vi "Save Instance VI to Polymorphic (strange poly vim saving).vi"(8 "error in (no error)":errorcluster, 10 "Polymorphic Label":string, 11 "SubVI Ref In":refnum<vi>) -> (0 "error out":errorcluster, 3 "Polymorphic VI":path)   [LabVIEW 2020]
uses:
  <vilib>/LabVIEW Icon API/LabVIEW Icon API.lvlib
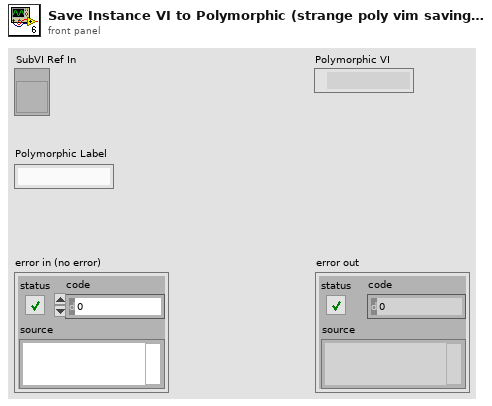
[diagram p1: front panel]
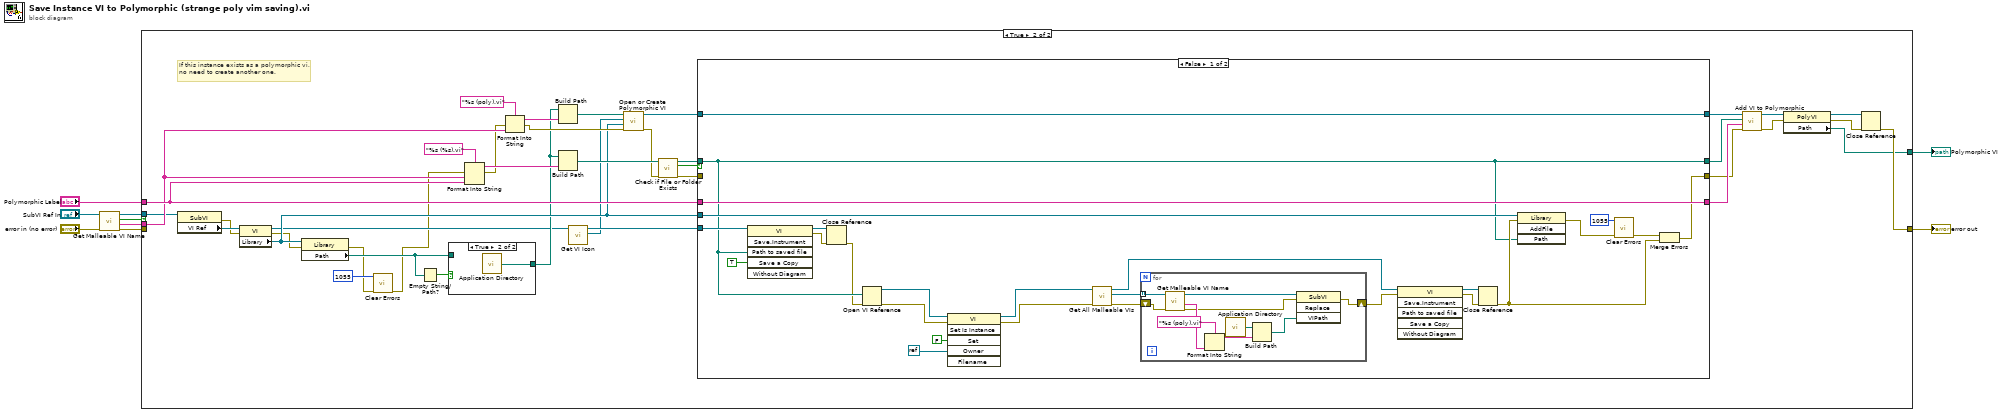
[diagram p0: block diagram]
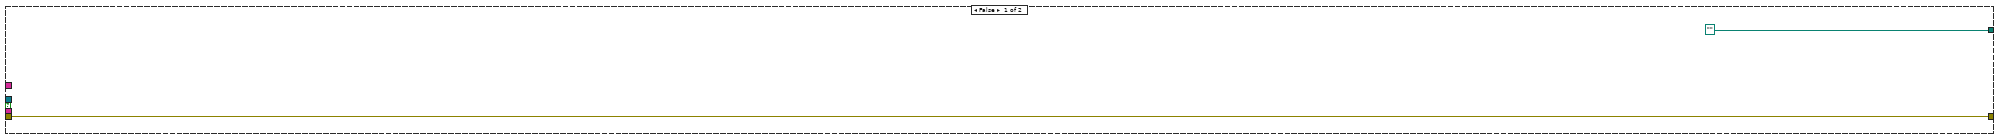
[diagram p2: hidden frame]
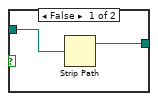
[diagram p3: hidden frame]
diagram:
  n1 = call "Get Malleable VI Name.vi"("error in (no error)"="error in (no error)", "SubVI Ref In"="SubVI Ref In") -> ("error out"=w3:errorcluster, "Name without extension"=w6:string, "Is Malleable VI?"=w7:bool, "SubVI Ref Out"=w8:refnum<vi>)  [unwired: 6 in]
  n2 = case shown="True" w7 {
    tunnel: w8 -> [_ w30]
    tunnel: w6 -> [_ w44]
    tunnel: "Polymorphic Label" -> [_ w46]
    tunnel: w3 -> [w11 _]
    tunnel: [w11 w31] -> w2
    tunnel: [path "" ("Path") w25] -> w1
    frame False {
    }
    frame True {
      # "If this instance exists as a polymorphic vi, no need to create another one."
      n3 = property class="SubVI"(reference=w30) -> (error out=w16:errorcluster, "VI Ref"=w20:refnum<vi>)  [unwired: 1 in, 1 out]
      n4 = property class="VI"(reference=w20, error in=w16) -> (reference out=w19:refnum<vi>, error out=w15:errorcluster, "Library"=w24:refnum<vi>)
      n5 = property class="Library"(reference=w24, error in=w15) -> (error out=w13:errorcluster, "Path"=w22:path)  [unwired: 1 out]
      n6 = call <vilib>:"Clear Errors.vi"("error in (no error)"=w13, "specific error code to clear (0: all)"=1055) -> ("error out"=w12:errorcluster)  [unwired: 4 in, 1 out]
      n7 = Empty String/Path?(string/path=w22) -> (empty?=w23:bool)
      n8 = case shown="True" w23 {
        tunnel: w22 -> [w52 _]
        tunnel: [w51 w53] -> w21
        frame False {
          n9 = Strip Path(path=w52) -> (stripped path=w51:path)  [unwired: 1 out]
        }
        frame True {
          n10 = call <vilib>:"Application Directory.vi"() -> ("Application Directory"=w53:path)
        }
      }
      n11 = Format Into String(format string="%s (%s).vi", error in=w12, w44, w46) -> (resulting string=w50:string, error out=w36:errorcluster)  [unwired: 1 in]
      n12 = Format Into String(format string="%s (poly).vi", error in=w36, w44) -> (resulting string=w42:string, error out=w35:errorcluster)  [unwired: 1 in]
      n13 = Build Path(base path=w21, name or relative path=w42) -> (appended path=w41:path)
      n14 = Build Path(base path=w21, name or relative path=w50) -> (appended path=w49:path)
      n15 = call <vilib>:"Get VI Icon.vi"("VI Refnum in"=w19) -> ("Icon"=w17:refnum<class "Icon.lvclass">, "VI Refnum out"=w18:refnum<vi>)  [unwired: 8 in, 1 out]
      n16 = call "Open or Create Polymorphic VI.vi"("error in (no error)"=w35, "Library"=w24, "Icon"=w17, "Polymorphic VI Path In"=w41) -> ("error out"=w34:errorcluster, "Polymorphic VI Refnum"=w40:refnum<vi>)  [unwired: 6 in]
      n17 = call <vilib>:"Check if File or Folder Exists.vi"("error in (no error)"=w34, "path"=w49) -> ("error out"=w33:errorcluster, "file or folder exists?"=w48:bool, "dup path"=w47:path)  [unwired: 7 in]
      n18 = case shown="False" w48 {
        tunnel: w47 -> [w61 w92]
        tunnel: w46 -> [w76 w91]
        tunnel: w40 -> [w77 w93]
        tunnel: [w77 w93] -> w39
        tunnel: [w61 w92] -> w38
        tunnel: [w76 w91] -> w37
        tunnel: w33 -> [_ w90]
        tunnel: [w66 w90] -> w32
        tunnel: w18 -> [w64 _]
        tunnel: w24 -> [w71 _]
        frame False {
          n19 = invoke class="VI" method="Save.Instrument"(reference=w64, "Path to saved file"=w61, "Save a Copy"=TRUE) -> (reference out=w63:refnum<vi>, error out=w62:errorcluster)  [unwired: 3 in, 4 out]
          n20 = Close Reference(reference=w63, error in (no error)=w62) -> (error out=w60:errorcluster)
          n21 = Open VI Reference(vi path=w61, error in (no error)=w60) -> (vi reference=w57:refnum<vi>, error out=w55:errorcluster)  [unwired: 4 in]
          n22 = invoke class="VI" method="Set Is Instance"(reference=w57, error in=w55, "Set"=FALSE, "Owner"=refnum<k0> refnum) -> (reference out=w56:refnum<vi>, error out=w54:errorcluster)  [unwired: 2 in, 4 out]
          n23 = call "Get All Malleable VIs.vi"("error in (no error)"=w54, "VI Ref In"=w56) -> ("error out"=w73:errorcluster, "Malleable VIs"=w75:refnum<vi>[], "VI Ref Out"=w74:refnum<vi>)  [unwired: 7 in]
          n24 = for {
            tunnel: w75 -> [w89] mode=indexing
            shift-right: [w80] -> w72
            shift-left: w73 -> [w82]
            n25 = call "Get Malleable VI Name.vi"("error in (no error)"=w82, "SubVI Ref In"=w89) -> ("error out"=w81:errorcluster, "Name without extension"=w88:string, "SubVI Ref Out"=w84:refnum<vi>)  [unwired: 6 in, 1 out]
            n26 = Format Into String(format string="%s (poly).vi", w88) -> (resulting string=w86:string)  [unwired: 2 in, 1 out]
            n27 = call <vilib>:"Application Directory.vi"() -> ("Application Directory"=w85:path)
            n28 = Build Path(base path=w85, name or relative path=w86) -> (appended path=w83:path)
            n29 = invoke class="SubVI" method="Replace"(reference=w84, error in=w81, "VIPath"=w83) -> (error out=w80:errorcluster)  [unwired: 1 in, 3 out]
          }
          n30 = invoke class="VI" method="Save.Instrument"(reference=w74, error in=w72) -> (reference out=w79:refnum<vi>, error out=w78:errorcluster)  [unwired: 4 in, 4 out]
          n31 = Close Reference(reference=w79, error in (no error)=w78) -> (error out=w67:errorcluster)
          n32 = invoke class="Library" method="AddFile"(reference=w71, error in=w67, "Path"=w61) -> (error out=w70:errorcluster)  [unwired: 1 in, 3 out]
          n33 = call <vilib>:"Clear Errors.vi"("error in (no error)"=w70, "specific error code to clear (0: all)"=1055) -> ("error out"=w68:errorcluster)  [unwired: 4 in, 1 out]
          n34 = Merge Errors(w68, w67) -> (w66:errorcluster)
        }
        frame True {
        }
      }
      n35 = call "Add VI to Polymorphic.vi"("error in (no error)"=w32, "Polymorphic Label"=w37, "Path"=w38, "Polymorphic VI Refnum In"=w39) -> ("error out"=w28:errorcluster, "Polymorphic VI Refnum Out"=w29:refnum<vi>)  [unwired: 6 in]
      n36 = property class="PolyVI"(reference=w29, error in=w28) -> (reference out=w26:refnum<vi>, error out=w27:errorcluster, "Path"=w25:path)
      n37 = Close Reference(reference=w26, error in (no error)=w27) -> (error out=w31:errorcluster)
    }
  }
  "error out" <- w2
  "Polymorphic VI" <- w1
